vi "Cross-Obstacle.vi"(6 "I2C Ref In":T1={"myRIO Reference"={"myRIO Model"=enum."Unknown", "myRIO Hardware Reference"={"Generic FPGA Reference"=refnum, "Allow multiple opens"=FALSE}}, "I2C Channels Enum"=enum."Not Connected", "I2C Configuration"={"I2C Transfer Rate"=enum."Fast mode (400 kbps)"}}, 7 "避障回數":enum16{"第一次避障", "第二次避障"}(ring), 8 "Error In":errorcluster, 9 "障礙物位置2":enum16{"1-1", "1-2", "2-1", "2-2"}(ring), 11 "障礙物位置":enum16{"障礙物一", "障礙物二"}(ring)) -> (0 "Error Out":errorcluster)   [LabVIEW 2019]
uses:
  <vilib>/myRIO/Instrument Drivers/Onboard IO/I2C/typedefs/I2C Reference.ctl
  <vilib>/myRIO/Common/Instrument Driver Framework/Utilities/typedefs/myRIO Generic Hardware Reference.ctl
  <vilib>/myRIO/Common/Instrument Driver Framework/Utilities/typedefs/Hardware Version Enum.ctl
  <vilib>/myRIO/Common/Instrument Driver Framework/Utilities/typedefs/myRIO v1.0 Reference.ctl
  <vilib>/myRIO/Common/Instrument Driver Framework/Utilities/typedefs/Generic FPGA Reference.ctl
  <vilib>/myRIO/Common/Instrument Driver Framework/myRIO v1.0/I2C/typedefs/I2C Channels Enum.ctl
  <vilib>/myRIO/Instrument Drivers/Onboard IO/I2C/typedefs/I2C Configuration.ctl
  <vilib>/myRIO/Instrument Drivers/Onboard IO/I2C/typedefs/I2C Transfer Rate.ctl
  <vilib>/myRIO/Instrument Drivers/Onboard IO/I2C/I2C.lvlib
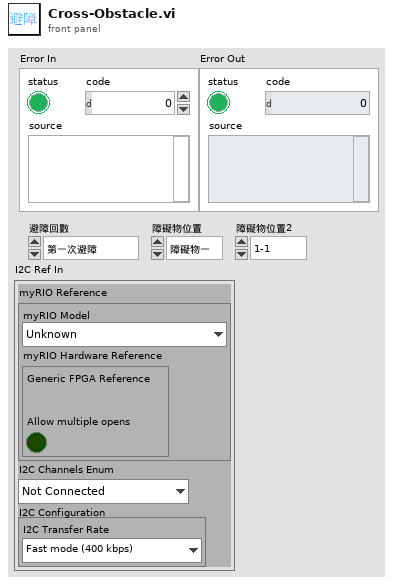
[diagram p1: front panel]
types:
  T1 = typedef "I2C.lvlib/I2C Reference.ctl" = cluster{"myRIO Reference":T2, "I2C Channels Enum":T6, "I2C Configuration":T7}
  T2 = typedef "myRIO Generic Hardware Reference.ctl" = cluster{"myRIO Model":T3, "myRIO Hardware Reference":T4}
  T3 = typedef "Hardware Version Enum.ctl" = enum16{"Unknown", "myRIO-1900", "myRIO-1950", "roboRIO", "NI ELVIS RIO CM", "ELVIS III"}
  T4 = typedef "myRIO v1.0 Reference.ctl" = cluster{"Generic FPGA Reference":T5, "Allow multiple opens":bool}
  T5 = typedef "Generic FPGA Reference.ctl" = refnum<k20>
  T6 = typedef "I2C Channels Enum.ctl" = enum16{"Not Connected", "A/I2C", "B/I2C", "I2C/I2C"}
  T7 = typedef "I2C.lvlib/I2C Configuration.ctl" = cluster{"I2C Transfer Rate":T8}
  T8 = typedef "I2C.lvlib/I2C Transfer Rate.ctl" = enum16{"Standard mode (100 kbps)", "Fast mode (400 kbps)"}
  T9 = enum16{"前", "後", "オ", "右", "無", "0", "1", "2", "3", "4", "5", "6", "7"}
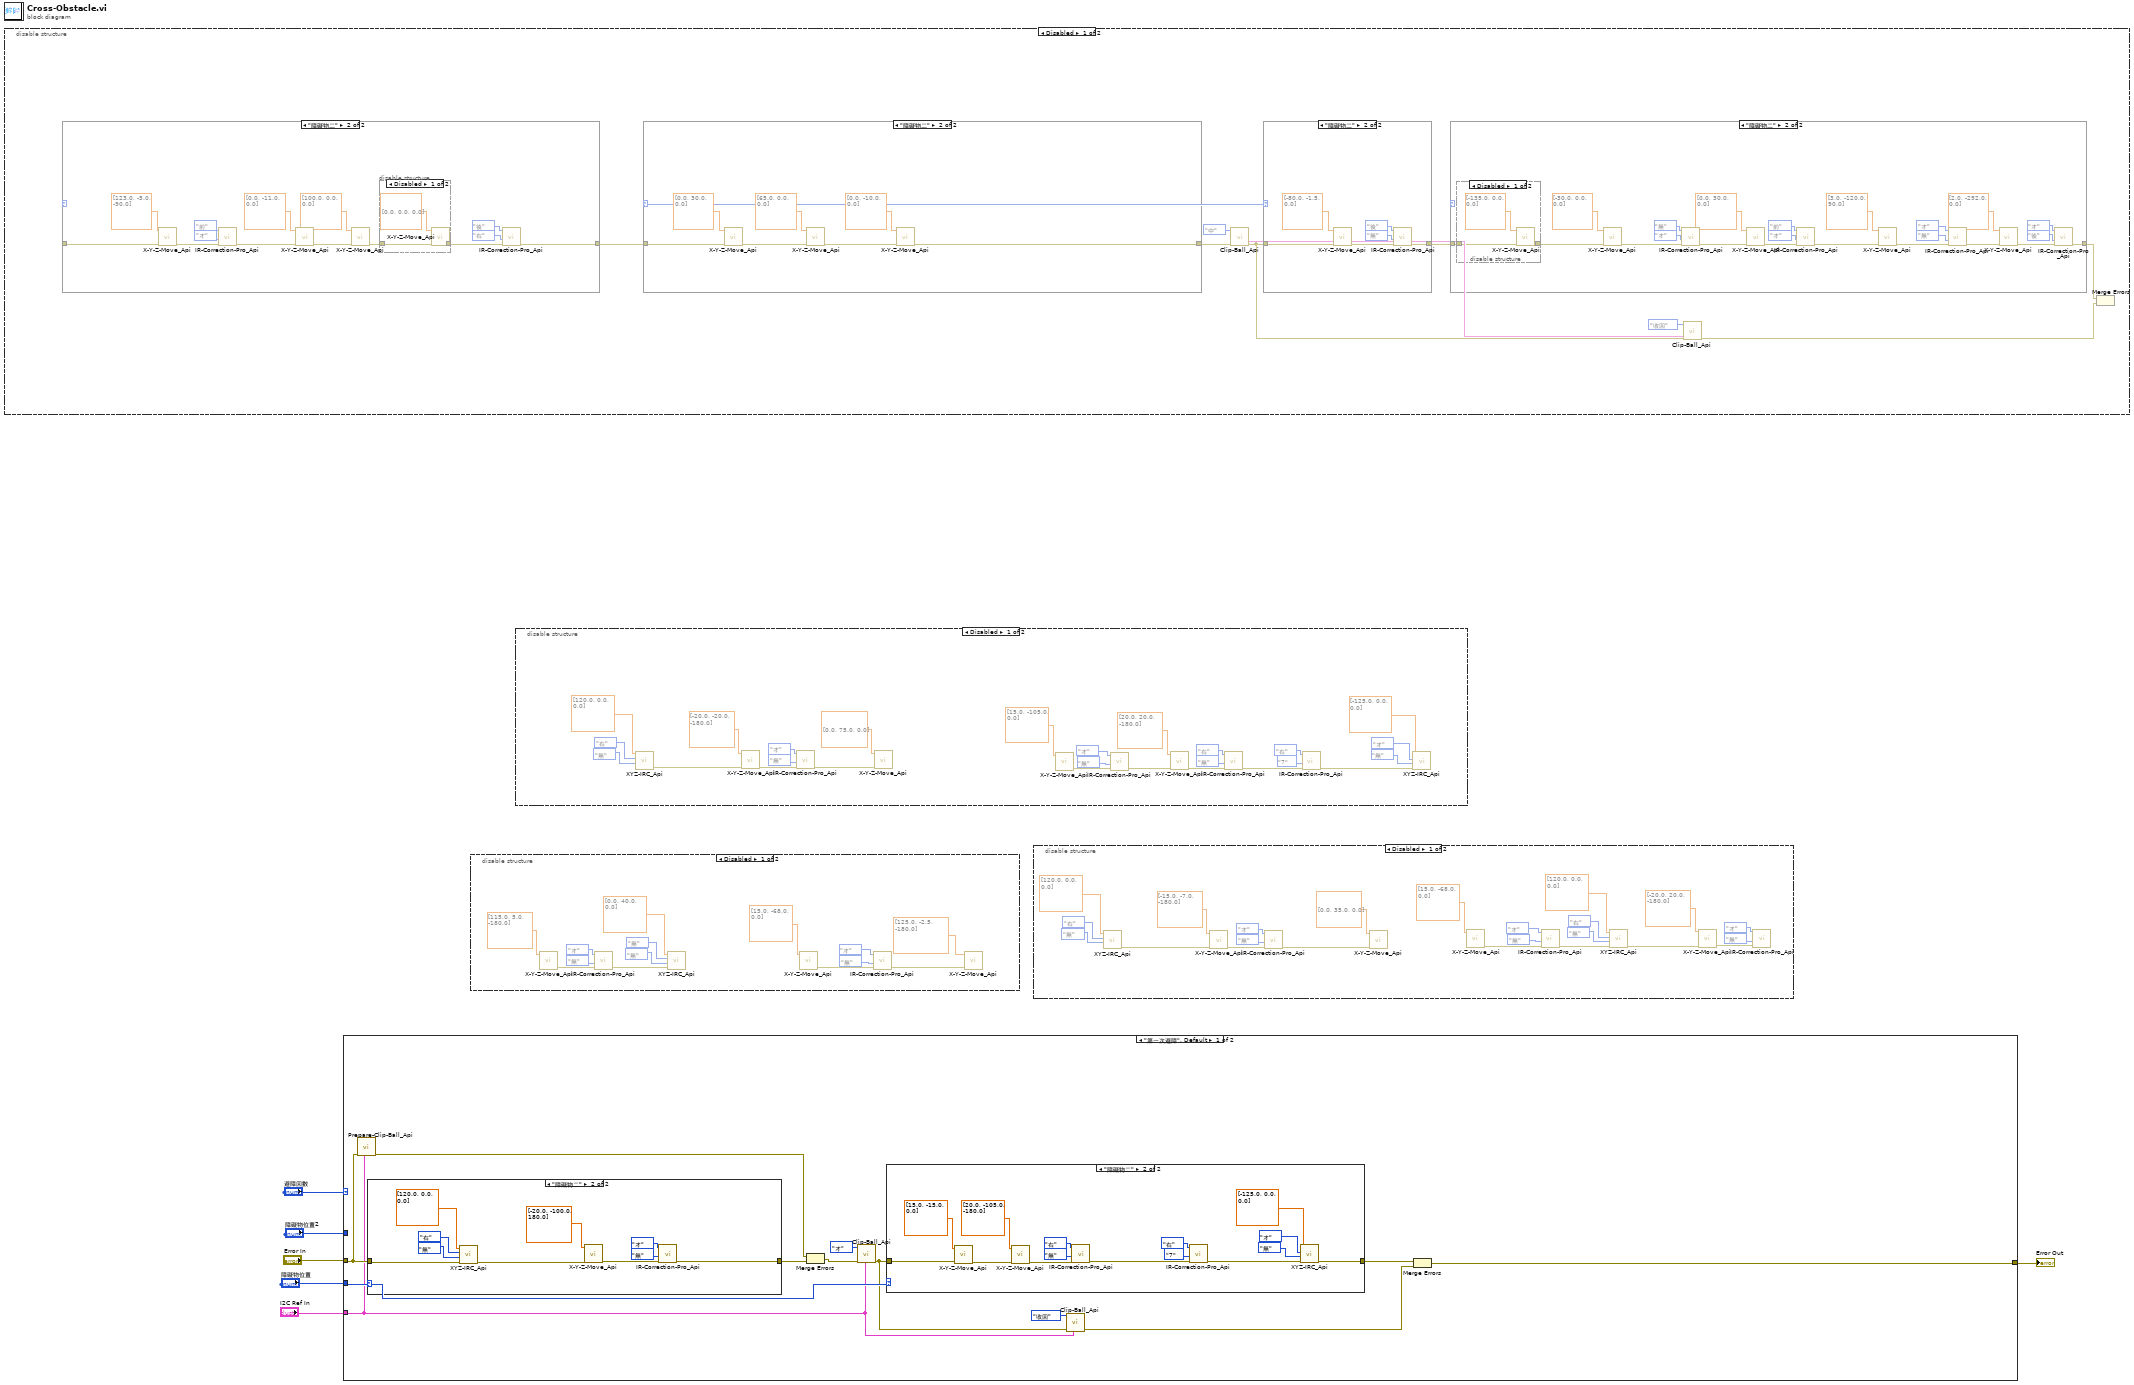
[diagram p0: block diagram]
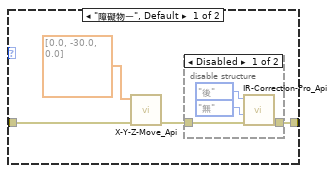
[diagram p5: hidden frame]
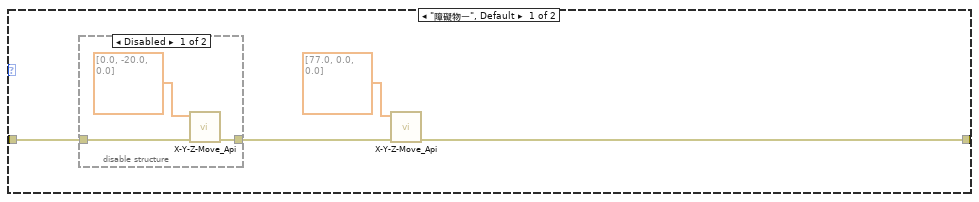
[diagram p7: hidden frame]
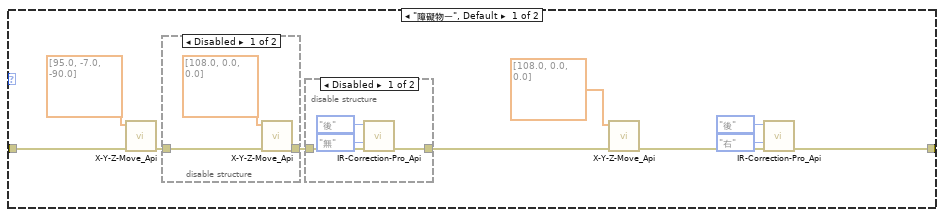
[diagram p9: hidden frame]
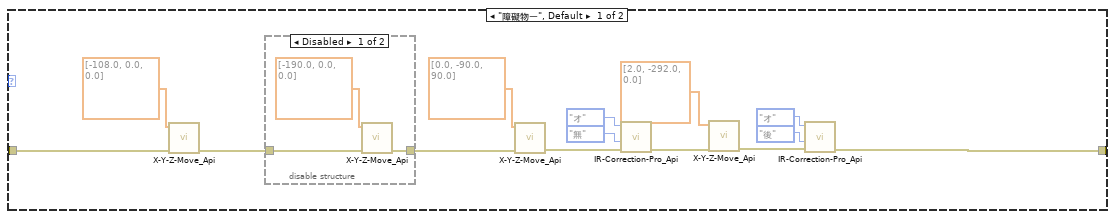
[diagram p13: hidden frame]
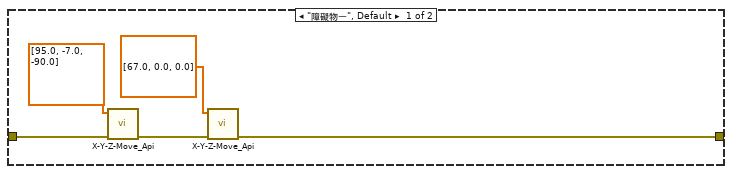
[diagram p17: hidden frame]
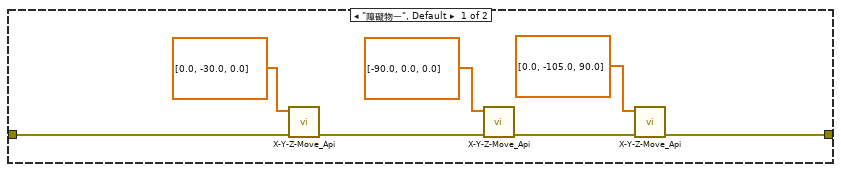
[diagram p18: hidden frame]
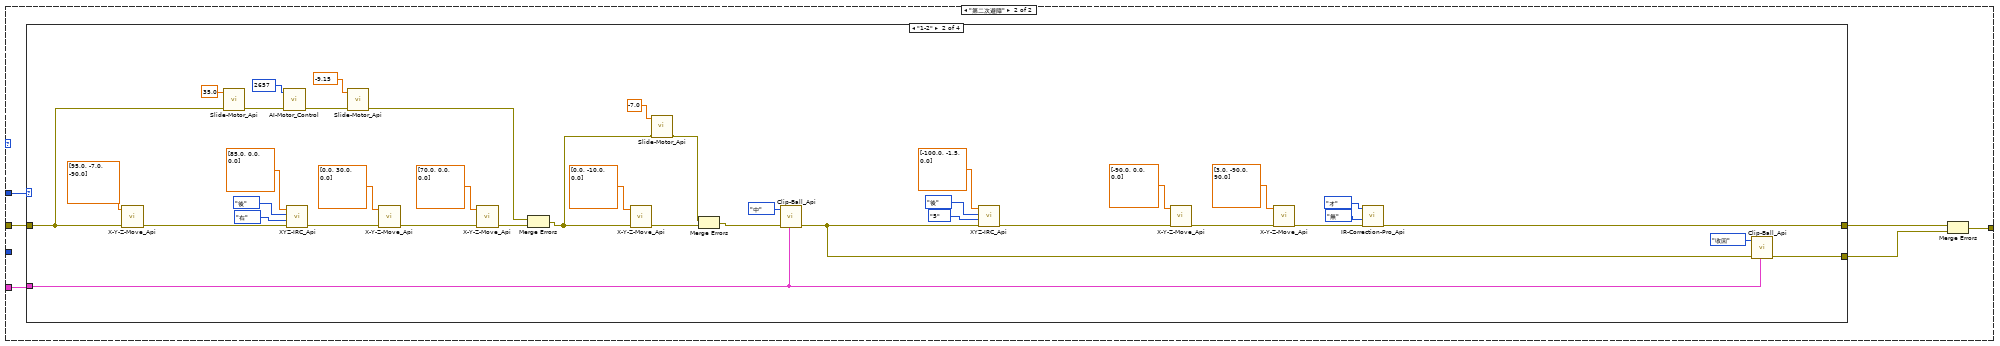
[diagram p19: hidden frame]
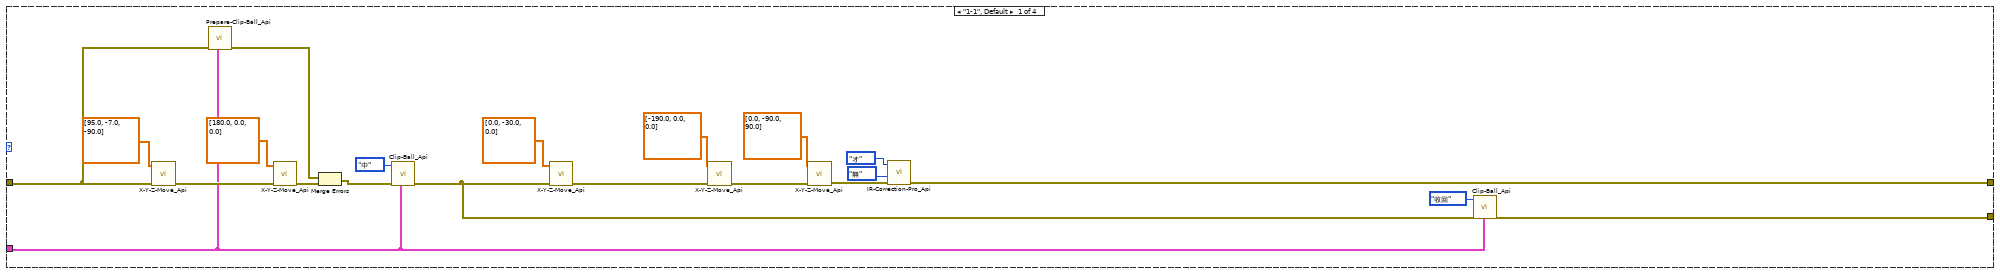
[diagram p20: hidden frame]
diagram:
  n1 = disable-structure shown="Disabled" {
    frame Disabled {
      n2 = case shown="\"障礙物二\"" {
        selector: _ -> [_ _]
        tunnel: [w56 w73] -> w16
        tunnel: [w50 w68] -> w15
        frame "障礙物一", Default {
          n3 = call "X-Y-Z-Move_Api.vi"("Error In"=w56, "X-Y-Z移動"=dbl[] [95.0, -7.0, -90.0]) -> ("Error Out"=w57:errorcluster)  [unwired: 8 in, 1 out]
          n4 = disable-structure shown="Disabled" {
            disable-tunnel: w57 -> [w60 w62]
            disable-tunnel: [w59 w62] -> w55
            frame Disabled {
              n5 = call "X-Y-Z-Move_Api.vi"("Error In"=w60, "X-Y-Z移動"=dbl[] [108.0, 0.0, 0.0]) -> ("Error Out"=w59:errorcluster)  [unwired: 8 in, 1 out]
            }
            frame Enabled {
            }
          }
          n6 = disable-structure shown="Disabled" {
            disable-tunnel: w55 -> [w66 w67]
            disable-tunnel: [w63 w67] -> w51
            frame Disabled {
              n7 = call "IR-Correction-Pro_Api.vi"("Error In"=w66, "副邊校正"=enum16{"前", "後", "オ", "右", "無"}."無", "主編校正"=enum16{"前", "後", "オ", "右", "無"}."後") -> ("Error Out"=w63:errorcluster)  [unwired: 8 in]
            }
            frame Enabled {
            }
          }
          n8 = call "X-Y-Z-Move_Api.vi"("Error In"=w51, "X-Y-Z移動"=dbl[] [108.0, 0.0, 0.0]) -> ("Error Out"=w54:errorcluster)  [unwired: 8 in, 1 out]
          n9 = call "IR-Correction-Pro_Api.vi"("Error In"=w54, "副邊校正"=enum16{"前", "後", "オ", "右", "無"}."右", "主編校正"=enum16{"前", "後", "オ", "右", "無"}."後") -> ("Error Out"=w50:errorcluster)  [unwired: 8 in]
        }
        frame "障礙物二" {
          n10 = call "X-Y-Z-Move_Api.vi"("Error In"=w73, "X-Y-Z移動"=dbl[] [123.0, -5.0, -90.0]) -> ("Error Out"=w79:errorcluster)  [unwired: 8 in, 1 out]
          n11 = call "IR-Correction-Pro_Api.vi"("Error In"=w79, "副邊校正"=enum16{"前", "後", "オ", "右", "無"}."オ", "主編校正"=enum16{"前", "後", "オ", "右", "無"}."前") -> ("Error Out"=w77:errorcluster)  [unwired: 8 in]
          n12 = call "X-Y-Z-Move_Api.vi"("Error In"=w77, "X-Y-Z移動"=dbl[] [0.0, -11.0, 0.0]) -> ("Error Out"=w74:errorcluster)  [unwired: 8 in, 1 out]
          n13 = call "X-Y-Z-Move_Api.vi"("Error In"=w74, "X-Y-Z移動"=dbl[] [100.0, 0.0, 0.0]) -> ("Error Out"=w75:errorcluster)  [unwired: 8 in, 1 out]
          n14 = disable-structure shown="Disabled" {
            disable-tunnel: w75 -> [w83 w85]
            disable-tunnel: [w82 w85] -> w69
            frame Disabled {
              n15 = call "X-Y-Z-Move_Api.vi"("Error In"=w83, "X-Y-Z移動"=dbl[] [0.0, 0.0, 0.0]) -> ("Error Out"=w82:errorcluster)  [unwired: 8 in, 1 out]
            }
            frame Enabled {
            }
          }
          n16 = call "IR-Correction-Pro_Api.vi"("Error In"=w69, "副邊校正"=enum16{"前", "後", "オ", "右", "無"}."右", "主編校正"=enum16{"前", "後", "オ", "右", "無"}."後") -> ("Error Out"=w68:errorcluster)  [unwired: 8 in]
        }
      }
      n17 = case shown="\"障礙物二\"" w17 {
        tunnel: w15 -> [w35 w47]
        tunnel: [w34 w42] -> w13
        frame "障礙物一", Default {
          n18 = disable-structure shown="Disabled" {
            disable-tunnel: [w39 w41] -> w36
            disable-tunnel: w35 -> [w38 w41]
            frame Disabled {
              n19 = call "X-Y-Z-Move_Api.vi"("Error In"=w38, "X-Y-Z移動"=dbl[] [0.0, -20.0, 0.0]) -> ("Error Out"=w39:errorcluster)  [unwired: 8 in, 1 out]
            }
            frame Enabled {
            }
          }
          n20 = call "X-Y-Z-Move_Api.vi"("Error In"=w36, "X-Y-Z移動"=dbl[] [77.0, 0.0, 0.0]) -> ("Error Out"=w34:errorcluster)  [unwired: 8 in, 1 out]
        }
        frame "障礙物二" {
          n21 = call "X-Y-Z-Move_Api.vi"("Error In"=w47, "X-Y-Z移動"=dbl[] [0.0, 30.0, 0.0]) -> ("Error Out"=w45:errorcluster)  [unwired: 8 in, 1 out]
          n22 = call "X-Y-Z-Move_Api.vi"("Error In"=w45, "X-Y-Z移動"=dbl[] [65.0, 0.0, 0.0]) -> ("Error Out"=w43:errorcluster)  [unwired: 8 in, 1 out]
          n23 = call "X-Y-Z-Move_Api.vi"("Error In"=w43, "X-Y-Z移動"=dbl[] [0.0, -10.0, 0.0]) -> ("Error Out"=w42:errorcluster)  [unwired: 8 in, 1 out]
        }
      }
      n24 = call "Clip-Ball_Api.vi"("Error In"=w13, "動作"=enum16{"オ", "中", "右", "收回"}."中") -> ("Error Out"=w10:errorcluster, "I2C Ref In"=w9:T1)  [unwired: 8 in]
      n25 = case shown="\"障礙物二\"" w17 {
        tunnel: w10 -> [w21 w32]
        tunnel: [w20 w28] -> w12
        frame "障礙物一", Default {
          n26 = call "X-Y-Z-Move_Api.vi"("Error In"=w21, "X-Y-Z移動"=dbl[] [0.0, -30.0, 0.0]) -> ("Error Out"=w19:errorcluster)  [unwired: 8 in, 1 out]
          n27 = disable-structure shown="Disabled" {
            disable-tunnel: [w24 w27] -> w20
            disable-tunnel: w19 -> [w23 w27]
            frame Disabled {
              n28 = call "IR-Correction-Pro_Api.vi"("Error In"=w23, "副邊校正"=enum16{"前", "後", "オ", "右", "無"}."無", "主編校正"=enum16{"前", "後", "オ", "右", "無"}."後") -> ("Error Out"=w24:errorcluster)  [unwired: 8 in]
            }
            frame Enabled {
            }
          }
        }
        frame "障礙物二" {
          n29 = call "X-Y-Z-Move_Api.vi"("Error In"=w32, "X-Y-Z移動"=dbl[] [-80.0, -1.5, 0.0]) -> ("Error Out"=w29:errorcluster)  [unwired: 8 in, 1 out]
          n30 = call "IR-Correction-Pro_Api.vi"("Error In"=w29, "副邊校正"=enum16{"前", "後", "オ", "右", "無"}."無", "主編校正"=enum16{"前", "後", "オ", "右", "無"}."後") -> ("Error Out"=w28:errorcluster)  [unwired: 8 in]
        }
      }
      n31 = case shown="\"障礙物二\"" w18 {
        tunnel: w12 -> [w86 w111]
        tunnel: [w89 w110] -> w8
        frame "障礙物一", Default {
          n32 = call "X-Y-Z-Move_Api.vi"("Error In"=w86, "X-Y-Z移動"=dbl[] [-108.0, 0.0, 0.0]) -> ("Error Out"=w87:errorcluster)  [unwired: 8 in, 1 out]
          n33 = disable-structure shown="Disabled" {
            disable-tunnel: w87 -> [w102 w103]
            disable-tunnel: [w100 w103] -> w98
            frame Disabled {
              n34 = call "X-Y-Z-Move_Api.vi"("Error In"=w102, "X-Y-Z移動"=dbl[] [-190.0, 0.0, 0.0]) -> ("Error Out"=w100:errorcluster)  [unwired: 8 in, 1 out]
            }
            frame Enabled {
            }
          }
          n35 = call "X-Y-Z-Move_Api.vi"("Error In"=w98, "X-Y-Z移動"=dbl[] [0.0, -90.0, 90.0]) -> ("Error Out"=w90:errorcluster)  [unwired: 8 in, 1 out]
          n36 = call "IR-Correction-Pro_Api.vi"("Error In"=w90, "副邊校正"=enum16{"前", "後", "オ", "右", "無"}."無", "主編校正"=enum16{"前", "後", "オ", "右", "無"}."オ") -> ("Error Out"=w92:errorcluster)  [unwired: 8 in]
          n37 = call "X-Y-Z-Move_Api.vi"("Error In"=w92, "X-Y-Z移動"=dbl[] [2.0, -292.0, 0.0]) -> ("Error Out"=w97:errorcluster)  [unwired: 8 in, 1 out]
          n38 = call "IR-Correction-Pro_Api.vi"("Error In"=w97, "副邊校正"=enum16{"前", "後", "オ", "右", "無"}."後", "主編校正"=enum16{"前", "後", "オ", "右", "無"}."オ") -> ("Error Out"=w89:errorcluster)  [unwired: 8 in]
        }
        frame "障礙物二" {
          n39 = disable-structure shown="Disabled" {
            disable-tunnel: w111 -> [w127 w129]
            disable-tunnel: [w126 w129] -> w104
            frame Disabled {
              n40 = call "X-Y-Z-Move_Api.vi"("Error In"=w127, "X-Y-Z移動"=dbl[] [-135.0, 0.0, 0.0]) -> ("Error Out"=w126:errorcluster)  [unwired: 8 in, 1 out]
            }
            frame Enabled {
            }
          }
          n41 = call "X-Y-Z-Move_Api.vi"("Error In"=w104, "X-Y-Z移動"=dbl[] [-30.0, 0.0, 0.0]) -> ("Error Out"=w105:errorcluster)  [unwired: 8 in, 1 out]
          n42 = call "IR-Correction-Pro_Api.vi"("Error In"=w105, "副邊校正"=enum16{"前", "後", "オ", "右", "無"}."オ", "主編校正"=enum16{"前", "後", "オ", "右", "無"}."無") -> ("Error Out"=w107:errorcluster)  [unwired: 8 in]
          n43 = call "X-Y-Z-Move_Api.vi"("Error In"=w107, "X-Y-Z移動"=dbl[] [0.0, 30.0, 0.0]) -> ("Error Out"=w114:errorcluster)  [unwired: 8 in, 1 out]
          n44 = call "IR-Correction-Pro_Api.vi"("Error In"=w114, "副邊校正"=enum16{"前", "後", "オ", "右", "無"}."オ", "主編校正"=enum16{"前", "後", "オ", "右", "無"}."前") -> ("Error Out"=w116:errorcluster)  [unwired: 8 in]
          n45 = call "X-Y-Z-Move_Api.vi"("Error In"=w116, "X-Y-Z移動"=dbl[] [3.0, -120.0, 90.0]) -> ("Error Out"=w117:errorcluster)  [unwired: 8 in, 1 out]
          n46 = call "IR-Correction-Pro_Api.vi"("Error In"=w117, "副邊校正"=enum16{"前", "後", "オ", "右", "無"}."無", "主編校正"=enum16{"前", "後", "オ", "右", "無"}."オ") -> ("Error Out"=w119:errorcluster)  [unwired: 8 in]
          n47 = call "X-Y-Z-Move_Api.vi"("Error In"=w119, "X-Y-Z移動"=dbl[] [2.0, -292.0, 0.0]) -> ("Error Out"=w124:errorcluster)  [unwired: 8 in, 1 out]
          n48 = call "IR-Correction-Pro_Api.vi"("Error In"=w124, "副邊校正"=enum16{"前", "後", "オ", "右", "無"}."後", "主編校正"=enum16{"前", "後", "オ", "右", "無"}."オ") -> ("Error Out"=w110:errorcluster)  [unwired: 8 in]
        }
      }
      n49 = call "Clip-Ball_Api.vi"("I2C Ref In"=w9, "Error In"=w10, "動作"=enum16{"オ", "中", "右", "收回"}."收回") -> ("Error Out"=w7:errorcluster)  [unwired: 8 in]
      n50 = Merge Errors(w8, w7) -> ()  [unwired: 1 out]
    }
    frame Enabled {
    }
  }
  n51 = case shown="\"第一次避障\", Default" "避障回數" {
    tunnel: "Error In" -> [w136 w184]
    tunnel: [w139 w180] -> w6
    tunnel: "障礙物位置" -> [w141 _]
    tunnel: "I2C Ref In" -> [w130 w181]
    tunnel: "障礙物位置2" -> [_ w183]
    frame "第一次避障", Default {
      n52 = call "Prepare-Clip-Ball_Api.vi"("I2C Ref In"=w130, "Error In"=w136) -> ("Error Out"=w133:errorcluster)  [unwired: 9 in]
      n53 = case shown="\"障礙物二\"" w141 {
        tunnel: w136 -> [w146 w152]
        tunnel: [w142 w148] -> w135
        frame "障礙物一", Default {
          n54 = call "X-Y-Z-Move_Api.vi"("Error In"=w146, "X-Y-Z移動"=dbl[] [95.0, -7.0, -90.0]) -> ("Error Out"=w143:errorcluster)  [unwired: 8 in, 1 out]
          n55 = call "X-Y-Z-Move_Api.vi"("Error In"=w143, "X-Y-Z移動"=dbl[] [67.0, 0.0, 0.0]) -> ("Error Out"=w142:errorcluster)  [unwired: 8 in, 1 out]
        }
        frame "障礙物二" {
          n56 = call "XYZ-IRC_Api.vi"("Error"=w152, "副邊校正"=T9."無", "主編校正"=enum16{"前", "後", "オ", "右", "無"}."右", "X-Y-Z移動"=dbl[] [120.0, 0.0, 0.0]) -> ("Error Out"=w147:errorcluster)  [unwired: 7 in]
          n57 = call "X-Y-Z-Move_Api.vi"("Error In"=w147, "X-Y-Z移動"=dbl[] [-20.0, -100.0, 180.0]) -> ("Error Out"=w149:errorcluster)  [unwired: 8 in, 1 out]
          n58 = call "IR-Correction-Pro_Api.vi"("Error In"=w149, "副邊校正"=T9."無", "主編校正"=enum16{"前", "後", "オ", "右", "無"}."オ") -> ("Error Out"=w148:errorcluster)  [unwired: 8 in]
        }
      }
      n59 = Merge Errors(w133, w135) -> (w134:errorcluster)
      n60 = call "Clip-Ball_Api.vi"("I2C Ref In"=w130, "Error In"=w134, "動作"=enum16{"オ", "中", "右", "收回", "合併"}."オ") -> ("Error Out"=w140:errorcluster)  [unwired: 8 in]
      n61 = case shown="\"障礙物二\"" w141 {
        tunnel: w140 -> [w157 w165]
        tunnel: [w161 w172] -> w138
        frame "障礙物一", Default {
          n62 = call "X-Y-Z-Move_Api.vi"("Error In"=w157, "X-Y-Z移動"=dbl[] [0.0, -30.0, 0.0]) -> ("Error Out"=w159:errorcluster)  [unwired: 8 in, 1 out]
          n63 = call "X-Y-Z-Move_Api.vi"("Error In"=w159, "X-Y-Z移動"=dbl[] [-90.0, 0.0, 0.0]) -> ("Error Out"=w158:errorcluster)  [unwired: 8 in, 1 out]
          n64 = call "X-Y-Z-Move_Api.vi"("Error In"=w158, "X-Y-Z移動"=dbl[] [0.0, -105.0, 90.0]) -> ("Error Out"=w161:errorcluster)  [unwired: 8 in, 1 out]
        }
        frame "障礙物二" {
          n65 = call "X-Y-Z-Move_Api.vi"("Error In"=w165, "X-Y-Z移動"=dbl[] [15.0, -15.0, 0.0]) -> ("Error Out"=w164:errorcluster)  [unwired: 8 in, 1 out]
          n66 = call "X-Y-Z-Move_Api.vi"("Error In"=w164, "X-Y-Z移動"=dbl[] [20.0, -105.0, -180.0]) -> ("Error Out"=w168:errorcluster)  [unwired: 8 in, 1 out]
          n67 = call "IR-Correction-Pro_Api.vi"("Error In"=w168, "副邊校正"=T9."無", "主編校正"=enum16{"前", "後", "オ", "右", "無"}."右") -> ("Error Out"=w167:errorcluster)  [unwired: 8 in]
          n68 = call "IR-Correction-Pro_Api.vi"("Error In"=w167, "副邊校正"=T9."7", "主編校正"=enum16{"前", "後", "オ", "右", "無"}."右") -> ("Error Out"=w171:errorcluster)  [unwired: 8 in]
          n69 = call "XYZ-IRC_Api.vi"("Error"=w171, "副邊校正"=T9."無", "主編校正"=enum16{"前", "後", "オ", "右", "無"}."オ", "X-Y-Z移動"=dbl[] [-125.0, 0.0, 0.0]) -> ("Error Out"=w172:errorcluster)  [unwired: 7 in]
        }
      }
      n70 = call "Clip-Ball_Api.vi"("I2C Ref In"=w130, "Error In"=w140, "動作"=enum16{"オ", "中", "右", "收回", "合併"}."收回") -> ("Error Out"=w137:errorcluster)  [unwired: 8 in]
      n71 = Merge Errors(w138, w137) -> (w139:errorcluster)
    }
    frame "第二次避障" {
      n72 = case shown="\"1-2\"" w183 {
        tunnel: w184 -> [w189 w211 w247 w301]
        tunnel: w181 -> [w185 w236 w278 w328]
        tunnel: [w193 w225 w261 w310] -> w182
        tunnel: [w195 w235 w276 w329] -> w179
        frame "1-1", Default {
          n73 = call "X-Y-Z-Move_Api.vi"("Error In"=w189, "X-Y-Z移動"=dbl[] [95.0, -7.0, -90.0]) -> ("Error Out"=w203:errorcluster)  [unwired: 8 in, 1 out]
          n74 = call "Prepare-Clip-Ball_Api.vi"("I2C Ref In"=w185, "Error In"=w189) -> ("Error Out"=w188:errorcluster)  [unwired: 9 in]
          n75 = call "X-Y-Z-Move_Api.vi"("Error In"=w203, "X-Y-Z移動"=dbl[] [180.0, 0.0, 0.0]) -> ("Error Out"=w191:errorcluster)  [unwired: 8 in, 1 out]
          n76 = Merge Errors(w188, w191) -> (w190:errorcluster)
          n77 = call "Clip-Ball_Api.vi"("I2C Ref In"=w185, "Error In"=w190, "動作"=enum16{"オ", "中", "右", "收回", "合併"}."中") -> ("Error Out"=w194:errorcluster)  [unwired: 8 in]
          n78 = call "X-Y-Z-Move_Api.vi"("Error In"=w194, "X-Y-Z移動"=dbl[] [0.0, -30.0, 0.0]) -> ("Error Out"=w200:errorcluster)  [unwired: 8 in, 1 out]
          n79 = call "X-Y-Z-Move_Api.vi"("Error In"=w200, "X-Y-Z移動"=dbl[] [-190.0, 0.0, 0.0]) -> ("Error Out"=w196:errorcluster)  [unwired: 8 in, 1 out]
          n80 = call "X-Y-Z-Move_Api.vi"("Error In"=w196, "X-Y-Z移動"=dbl[] [0.0, -90.0, 90.0]) -> ("Error Out"=w197:errorcluster)  [unwired: 8 in, 1 out]
          n81 = call "IR-Correction-Pro_Api.vi"("Error In"=w197, "副邊校正"=T9."無", "主編校正"=enum16{"前", "後", "オ", "右", "無"}."オ") -> ("Error Out"=w193:errorcluster)  [unwired: 8 in]
          n82 = call "Clip-Ball_Api.vi"("I2C Ref In"=w185, "Error In"=w194, "動作"=enum16{"オ", "中", "右", "收回", "合併"}."收回") -> ("Error Out"=w195:errorcluster)  [unwired: 8 in]
        }
        frame "1-2" {
          n83 = call "X-Y-Z-Move_Api.vi"("Error In"=w211, "X-Y-Z移動"=dbl[] [95.0, -7.0, -90.0]) -> ("Error Out"=w232:errorcluster)  [unwired: 8 in, 1 out]
          n84 = call "Slide-Motor_Api.vi"("Error In"=w211, "移動距離"=35.0) -> ("Error Out"=w214:errorcluster)  [unwired: 9 in]
          n85 = call "AI-Motor_Control.vi"("Error In"=w214, "目標位置(0~4095)"=u16 2657) -> ("Error Out"=w213:errorcluster)  [unwired: 9 in]
          n86 = call "XYZ-IRC_Api.vi"("Error"=w232, "副邊校正"=T9."右", "主編校正"=enum16{"前", "後", "オ", "右", "無"}."後", "X-Y-Z移動"=dbl[] [85.0, 0.0, 0.0]) -> ("Error Out"=w231:errorcluster)  [unwired: 7 in]
          n87 = call "Slide-Motor_Api.vi"("Error In"=w213, "移動距離"=-9.15) -> ("Error Out"=w212:errorcluster)  [unwired: 9 in]
          n88 = call "X-Y-Z-Move_Api.vi"("Error In"=w231, "X-Y-Z移動"=dbl[] [0.0, 30.0, 0.0]) -> ("Error Out"=w240:errorcluster)  [unwired: 8 in, 1 out]
          n89 = call "X-Y-Z-Move_Api.vi"("Error In"=w240, "X-Y-Z移動"=dbl[] [70.0, 0.0, 0.0]) -> ("Error Out"=w218:errorcluster)  [unwired: 8 in, 1 out]
          n90 = Merge Errors(w212, w218) -> (w208:errorcluster)
          n91 = call "X-Y-Z-Move_Api.vi"("Error In"=w208, "X-Y-Z移動"=dbl[] [0.0, -10.0, 0.0]) -> ("Error Out"=w220:errorcluster)  [unwired: 8 in, 1 out]
          n92 = call "Slide-Motor_Api.vi"("Error In"=w208, "移動距離"=-7.0) -> ("Error Out"=w209:errorcluster)  [unwired: 9 in]
          n93 = Merge Errors(w209, w220) -> (w219:errorcluster)
          n94 = call "Clip-Ball_Api.vi"("I2C Ref In"=w236, "Error In"=w219, "動作"=enum16{"オ", "中", "右", "收回", "合併"}."中") -> ("Error Out"=w224:errorcluster)  [unwired: 8 in]
          n95 = call "XYZ-IRC_Api.vi"("Error"=w224, "副邊校正"=T9."5", "主編校正"=enum16{"前", "後", "オ", "右", "無"}."後", "X-Y-Z移動"=dbl[] [-100.0, -1.5, 0.0]) -> ("Error Out"=w227:errorcluster)  [unwired: 7 in]
          n96 = call "X-Y-Z-Move_Api.vi"("Error In"=w227, "X-Y-Z移動"=dbl[] [-90.0, 0.0, 0.0]) -> ("Error Out"=w226:errorcluster)  [unwired: 8 in, 1 out]
          n97 = call "X-Y-Z-Move_Api.vi"("Error In"=w226, "X-Y-Z移動"=dbl[] [3.0, -90.0, 90.0]) -> ("Error Out"=w237:errorcluster)  [unwired: 8 in, 1 out]
          n98 = call "IR-Correction-Pro_Api.vi"("Error In"=w237, "副邊校正"=T9."無", "主編校正"=enum16{"前", "後", "オ", "右", "無"}."オ") -> ("Error Out"=w225:errorcluster)  [unwired: 8 in]
          n99 = call "Clip-Ball_Api.vi"("I2C Ref In"=w236, "Error In"=w224, "動作"=enum16{"オ", "中", "右", "收回", "合併"}."收回") -> ("Error Out"=w235:errorcluster)  [unwired: 8 in]
        }
        frame "2-1" {
          n100 = call "X-Y-Z-Move_Api.vi"("Error In"=w247, "X-Y-Z移動"=dbl[] [123.0, -5.0, -90.0]) -> ("Error Out"=w286:errorcluster)  [unwired: 8 in, 1 out]
          n101 = call "IR-Correction-Pro_Api.vi"("Error In"=w286, "副邊校正"=T9."無", "主編校正"=enum16{"前", "後", "オ", "右", "無"}."前") -> ("Error Out"=w256:errorcluster)  [unwired: 8 in]
          n102 = call "XYZ-IRC_Api.vi"("Error"=w256, "副邊校正"=T9."右", "主編校正"=enum16{"前", "後", "オ", "右", "無"}."無", "X-Y-Z移動"=dbl[] [0.0, 10.0, 0.0]) -> ("Error Out"=w273:errorcluster)  [unwired: 7 in]
          n103 = call "X-Y-Z-Move_Api.vi"("Error In"=w273, "X-Y-Z移動"=dbl[] [0.0, -18.0, 0.0]) -> ("Error Out"=w270:errorcluster)  [unwired: 8 in, 1 out]
          n104 = call "Prepare-Clip-Ball_Api.vi"("Error In"=w247) -> ("Error Out"=w248:errorcluster)  [unwired: 10 in]
          n105 = call "XYZ-IRC_Api.vi"("Error"=w270, "副邊校正"=T9."無", "主編校正"=enum16{"前", "後", "オ", "右", "無"}."後", "X-Y-Z移動"=dbl[] [65.0, 0.0, 0.0]) -> ("Error Out"=w269:errorcluster)  [unwired: 7 in]
          n106 = call "X-Y-Z-Move_Api.vi"("Error In"=w269, "X-Y-Z移動"=dbl[] [70.0, 0.0, 0.0]) -> ("Error Out"=w250:errorcluster)  [unwired: 8 in, 1 out]
          n107 = Merge Errors(w248, w250) -> (w249:errorcluster)
          n108 = call "Clip-Ball_Api.vi"("I2C Ref In"=w278, "Error In"=w249, "動作"=enum16{"オ", "中", "右", "收回", "合併"}."中") -> ("Error Out"=w277:errorcluster)  [unwired: 8 in]
          n109 = call "X-Y-Z-Move_Api.vi"("Error In"=w277, "X-Y-Z移動"=dbl[] [0.0, -30.0, 0.0]) -> ("Error Out"=w266:errorcluster)  [unwired: 8 in, 1 out]
          n110 = call "XYZ-IRC_Api.vi"("Error"=w266, "副邊校正"=T9."オ", "主編校正"=enum16{"前", "後", "オ", "右", "無"}."無", "X-Y-Z移動"=dbl[] [-108.0, 0.0, 0.0]) -> ("Error Out"=w259:errorcluster)  [unwired: 7 in]
          n111 = call "X-Y-Z-Move_Api.vi"("Error In"=w259, "X-Y-Z移動"=dbl[] [0.0, 35.0, 0.0]) -> ("Error Out"=w258:errorcluster)  [unwired: 8 in, 1 out]
          n112 = call "XYZ-IRC_Api.vi"("Error"=w258, "副邊校正"=T9."オ", "主編校正"=enum16{"前", "後", "オ", "右", "無"}."前", "X-Y-Z移動"=dbl[] [-40.0, 0.0, 0.0]) -> ("Error Out"=w263:errorcluster)  [unwired: 7 in]
          n113 = disable-structure shown="Disabled" {
            disable-tunnel: w263 -> [w289 w291]
            disable-tunnel: [w288 w291] -> w262
            frame Disabled {
              n114 = call "X-Y-Z-Move_Api.vi"("Error In"=w289, "X-Y-Z移動"=dbl[] [18.0, 0.0, 0.0]) -> ("Error Out"=w288:errorcluster)  [unwired: 8 in, 1 out]
            }
            frame Enabled {
            }
          }
          n115 = call "X-Y-Z-Move_Api.vi"("Error In"=w262, "X-Y-Z移動"=dbl[] [3.0, -120.0, 90.0]) -> ("Error Out"=w279:errorcluster)  [unwired: 8 in, 1 out]
          n116 = call "IR-Correction-Pro_Api.vi"("Error In"=w279, "副邊校正"=T9."無", "主編校正"=enum16{"前", "後", "オ", "右", "無"}."オ") -> ("Error Out"=w261:errorcluster)  [unwired: 8 in]
          n117 = call "Clip-Ball_Api.vi"("I2C Ref In"=w278, "Error In"=w277, "動作"=enum16{"オ", "中", "右", "收回", "合併"}."收回") -> ("Error Out"=w276:errorcluster)  [unwired: 8 in]
        }
        frame "2-2" {
          n118 = call "X-Y-Z-Move_Api.vi"("Error In"=w301, "X-Y-Z移動"=dbl[] [123.0, -5.0, -90.0]) -> ("Error Out"=w309:errorcluster)  [unwired: 8 in, 1 out]
          n119 = call "IR-Correction-Pro_Api.vi"("Error In"=w309, "副邊校正"=T9."無", "主編校正"=enum16{"前", "後", "オ", "右", "無"}."前") -> ("Error Out"=w324:errorcluster)  [unwired: 8 in]
          n120 = call "XYZ-IRC_Api.vi"("Error"=w324, "副邊校正"=T9."右", "主編校正"=enum16{"前", "後", "オ", "右", "無"}."無", "X-Y-Z移動"=dbl[] [0.0, 10.0, 0.0]) -> ("Error Out"=w323:errorcluster)  [unwired: 7 in]
          n121 = call "X-Y-Z-Move_Api.vi"("Error In"=w323, "X-Y-Z移動"=dbl[] [7.0, -20.0, 0.0]) -> ("Error Out"=w320:errorcluster)  [unwired: 8 in, 1 out]
          n122 = call "Prepare-Clip-Ball_Api.vi"("Error In"=w301) -> ("Error Out"=w298:errorcluster)  [unwired: 10 in]
          n123 = call "XYZ-IRC_Api.vi"("Error"=w320, "副邊校正"=T9."右", "主編校正"=enum16{"前", "後", "オ", "右", "無"}."後", "X-Y-Z移動"=dbl[] [40.0, 0.0, 0.0]) -> ("Error Out"=w319:errorcluster)  [unwired: 7 in]
          n124 = call "X-Y-Z-Move_Api.vi"("Error In"=w319, "X-Y-Z移動"=dbl[] [0.0, 30.0, 0.0]) -> ("Error Out"=w335:errorcluster)  [unwired: 8 in, 1 out]
          n125 = call "X-Y-Z-Move_Api.vi"("Error In"=w335, "X-Y-Z移動"=dbl[] [65.0, 0.0, 0.0]) -> ("Error Out"=w333:errorcluster)  [unwired: 8 in, 1 out]
          n126 = call "X-Y-Z-Move_Api.vi"("Error In"=w333, "X-Y-Z移動"=dbl[] [0.0, -10.0, 0.0]) -> ("Error Out"=w300:errorcluster)  [unwired: 8 in, 1 out]
          n127 = Merge Errors(w298, w300) -> (w299:errorcluster)
          n128 = call "Clip-Ball_Api.vi"("I2C Ref In"=w328, "Error In"=w299, "動作"=enum16{"オ", "中", "右", "收回", "合併"}."中") -> ("Error Out"=w316:errorcluster)  [unwired: 8 in]
          n129 = call "XYZ-IRC_Api.vi"("Error"=w316, "副邊校正"=T9."無", "主編校正"=enum16{"前", "後", "オ", "右", "無"}."後", "X-Y-Z移動"=dbl[] [-90.0, -1.5, 0.0]) -> ("Error Out"=w313:errorcluster)  [unwired: 7 in]
          n130 = call "XYZ-IRC_Api.vi"("Error"=w313, "副邊校正"=T9."オ", "主編校正"=enum16{"前", "後", "オ", "右", "無"}."無", "X-Y-Z移動"=dbl[] [-30.0, 0.0, 0.0]) -> ("Error Out"=w295:errorcluster)  [unwired: 7 in]
          n131 = call "X-Y-Z-Move_Api.vi"("Error In"=w295, "X-Y-Z移動"=dbl[] [0.0, 35.0, 0.0]) -> ("Error Out"=w294:errorcluster)  [unwired: 8 in, 1 out]
          n132 = call "XYZ-IRC_Api.vi"("Error"=w294, "副邊校正"=T9."オ", "主編校正"=enum16{"前", "後", "オ", "右", "無"}."前", "X-Y-Z移動"=dbl[] [-20.0, 0.0, 0.0]) -> ("Error Out"=w297:errorcluster)  [unwired: 7 in]
          n133 = call "Clip-Ball_Api.vi"("I2C Ref In"=w328, "Error In"=w316, "動作"=enum16{"オ", "中", "右", "收回", "合併"}."收回") -> ("Error Out"=w329:errorcluster)  [unwired: 8 in]
          n134 = call "X-Y-Z-Move_Api.vi"("Error In"=w297, "X-Y-Z移動"=dbl[] [3.0, -120.0, 90.0]) -> ("Error Out"=w330:errorcluster)  [unwired: 8 in, 1 out]
          n135 = call "IR-Correction-Pro_Api.vi"("Error In"=w330, "副邊校正"=T9."無", "主編校正"=enum16{"前", "後", "オ", "右", "無"}."オ") -> ("Error Out"=w310:errorcluster)  [unwired: 8 in]
        }
      }
      n136 = Merge Errors(w182, w179) -> (w180:errorcluster)
    }
  }
  "Error Out" <- w6
  n137 = disable-structure shown="Disabled" {
    frame Disabled {
      n138 = call "X-Y-Z-Move_Api.vi"("X-Y-Z移動"=dbl[] [115.0, 5.0, -180.0]) -> ("Error Out"=w351:errorcluster)  [unwired: 9 in, 1 out]
      n139 = call "IR-Correction-Pro_Api.vi"("Error In"=w351, "副邊校正"=T9."無", "主編校正"=enum16{"前", "後", "オ", "右", "無"}."オ") -> ("Error Out"=w349:errorcluster)  [unwired: 8 in]
      n140 = call "XYZ-IRC_Api.vi"("Error"=w349, "副邊校正"=T9."無", "主編校正"=enum16{"前", "後", "オ", "右", "無"}."無", "X-Y-Z移動"=dbl[] [0.0, 40.0, 0.0]) -> ()  [unwired: 7 in, 1 out]
      n141 = call "X-Y-Z-Move_Api.vi"("X-Y-Z移動"=dbl[] [15.0, -68.0, 0.0]) -> ("Error Out"=w343:errorcluster)  [unwired: 9 in, 1 out]
      n142 = call "IR-Correction-Pro_Api.vi"("Error In"=w343, "副邊校正"=T9."無", "主編校正"=enum16{"前", "後", "オ", "右", "無"}."オ") -> ("Error Out"=w342:errorcluster)  [unwired: 8 in]
      n143 = call "X-Y-Z-Move_Api.vi"("Error In"=w342, "X-Y-Z移動"=dbl[] [125.0, -2.5, -180.0]) -> ()  [unwired: 8 in, 2 out]
    }
    frame Enabled {
    }
  }
  n144 = disable-structure shown="Disabled" {
    frame Disabled {
      n145 = call "XYZ-IRC_Api.vi"("副邊校正"=T9."無", "主編校正"=enum16{"前", "後", "オ", "右", "無"}."右", "X-Y-Z移動"=dbl[] [120.0, 0.0, 0.0]) -> ("Error Out"=w374:errorcluster, "Error"=w371:errorcluster)  [unwired: 7 in]
      n146 = call "X-Y-Z-Move_Api.vi"("Error In"=w374, "X-Y-Z移動"=dbl[] [-20.0, -20.0, -180.0]) -> ("Error Out"=w376:errorcluster)  [unwired: 8 in, 1 out]
      n147 = call "IR-Correction-Pro_Api.vi"("Error In"=w376, "副邊校正"=T9."無", "主編校正"=enum16{"前", "後", "オ", "右", "無"}."オ") -> ("Error Out"=w372:errorcluster)  [unwired: 8 in]
      n148 = call "X-Y-Z-Move_Api.vi"("Error In"=w372, "X-Y-Z移動"=dbl[] [0.0, 75.0, 0.0]) -> ()  [unwired: 8 in, 2 out]
      n149 = call "X-Y-Z-Move_Api.vi"("X-Y-Z移動"=dbl[] [15.0, -105.0, 0.0]) -> ("Error Out"=w369:errorcluster, "Error In"=w366:errorcluster)  [unwired: 8 in, 1 out]
      n150 = call "IR-Correction-Pro_Api.vi"("Error In"=w369, "副邊校正"=T9."無", "主編校正"=enum16{"前", "後", "オ", "右", "無"}."オ") -> ("Error Out"=w359:errorcluster)  [unwired: 8 in]
      n151 = call "X-Y-Z-Move_Api.vi"("Error In"=w359, "X-Y-Z移動"=dbl[] [20.0, 20.0, -180.0]) -> ("Error Out"=w358:errorcluster)  [unwired: 8 in, 1 out]
      n152 = call "IR-Correction-Pro_Api.vi"("Error In"=w358, "副邊校正"=T9."無", "主編校正"=enum16{"前", "後", "オ", "右", "無"}."右") -> ("Error Out"=w361:errorcluster)  [unwired: 8 in]
      n153 = call "IR-Correction-Pro_Api.vi"("Error In"=w361, "副邊校正"=T9."7", "主編校正"=enum16{"前", "後", "オ", "右", "無"}."右") -> ("Error Out"=w354:errorcluster)  [unwired: 8 in]
      n154 = call "XYZ-IRC_Api.vi"("Error"=w354, "副邊校正"=T9."無", "主編校正"=enum16{"前", "後", "オ", "右", "無"}."オ", "X-Y-Z移動"=dbl[] [-125.0, 0.0, 0.0]) -> ()  [unwired: 7 in, 1 out]
    }
    frame Enabled {
    }
  }
  n155 = disable-structure shown="Disabled" {
    frame Disabled {
      n156 = call "XYZ-IRC_Api.vi"("副邊校正"=T9."無", "主編校正"=enum16{"前", "後", "オ", "右", "無"}."右", "X-Y-Z移動"=dbl[] [120.0, 0.0, 0.0]) -> ("Error Out"=w397:errorcluster)  [unwired: 8 in]
      n157 = call "X-Y-Z-Move_Api.vi"("Error In"=w397, "X-Y-Z移動"=dbl[] [-15.0, -7.0, -180.0]) -> ("Error Out"=w399:errorcluster)  [unwired: 8 in, 1 out]
      n158 = call "IR-Correction-Pro_Api.vi"("Error In"=w399, "副邊校正"=T9."無", "主編校正"=enum16{"前", "後", "オ", "右", "無"}."オ") -> ("Error Out"=w395:errorcluster)  [unwired: 8 in]
      n159 = call "X-Y-Z-Move_Api.vi"("Error In"=w395, "X-Y-Z移動"=dbl[] [0.0, 35.0, 0.0]) -> ()  [unwired: 8 in, 2 out]
      n160 = call "X-Y-Z-Move_Api.vi"("X-Y-Z移動"=dbl[] [15.0, -68.0, 0.0]) -> ("Error Out"=w393:errorcluster)  [unwired: 9 in, 1 out]
      n161 = call "IR-Correction-Pro_Api.vi"("Error In"=w393, "副邊校正"=T9."無", "主編校正"=enum16{"前", "後", "オ", "右", "無"}."オ") -> ("Error Out"=w382:errorcluster)  [unwired: 8 in]
      n162 = call "XYZ-IRC_Api.vi"("Error"=w382, "副邊校正"=T9."無", "主編校正"=enum16{"前", "後", "オ", "右", "無"}."右", "X-Y-Z移動"=dbl[] [120.0, 0.0, 0.0]) -> ("Error Out"=w383:errorcluster)  [unwired: 7 in]
      n163 = call "X-Y-Z-Move_Api.vi"("Error In"=w383, "X-Y-Z移動"=dbl[] [-20.0, 20.0, -180.0]) -> ("Error Out"=w385:errorcluster)  [unwired: 8 in, 1 out]
      n164 = call "IR-Correction-Pro_Api.vi"("Error In"=w385, "副邊校正"=T9."無", "主編校正"=enum16{"前", "後", "オ", "右", "無"}."オ") -> ()  [unwired: 8 in, 1 out]
    }
    frame Enabled {
    }
  }
